vi "Write Sheet3 Data.vi"(0 "Cal Path":path, 5 "Actual Table 1":string[][](array[string]), 7 "Dev Table 1":string[][](array[string]), 9 "Dev Table 2":string[][](array[string]), 11 "Cal Point":i32) -> ()   [LabVIEW 2013]
uses:
  Type Defs/Excel Driver Operator Type Def.ctl
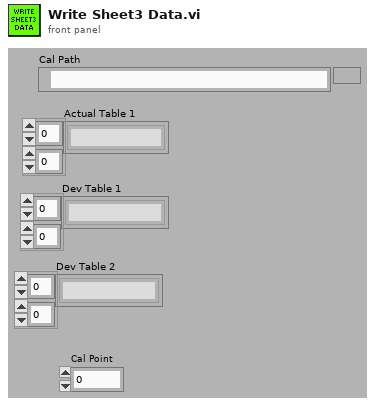
[diagram p1: front panel]
types:
  T1 = typedef "Excel Driver Operator Type Def.ctl" = enum16{"Open", "Close", "Search for String", "GetUsedRange", "Read Range", "Read Cell", "Set Range", "Set Cell"}
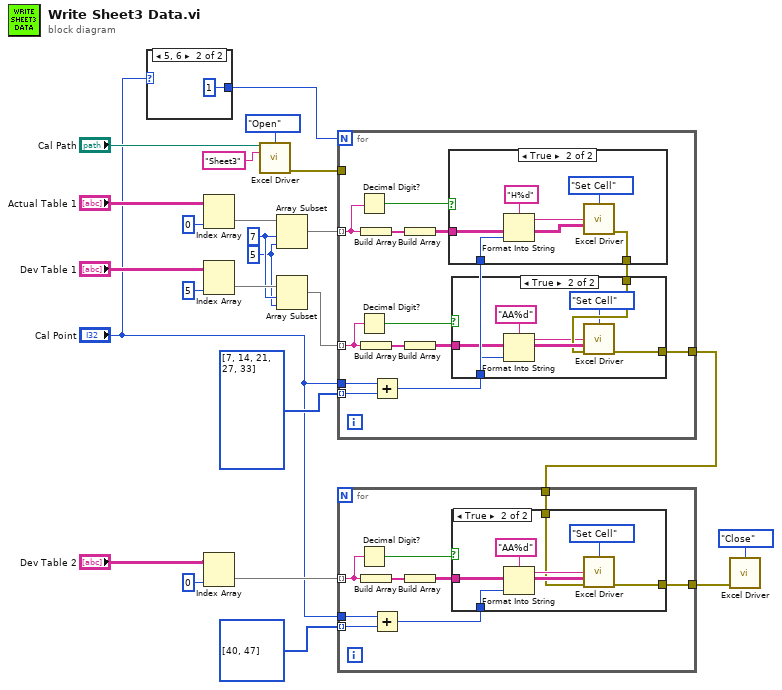
[diagram p0: block diagram]
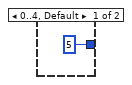
[diagram p2: hidden frame]
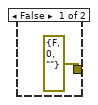
[diagram p3: hidden frame]
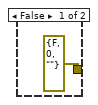
[diagram p4: hidden frame]
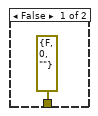
[diagram p5: hidden frame]
diagram:
  w12 = 5 ("length")
  w13 = 7 ("index")
  n1 = case shown="5, 6" "Cal Point" {
    tunnel: [5 1] -> w1
    frame 0..4, Default {
    }
    frame 5, 6 {
    }
  }
  n2 = Index Array(array="Actual Table 1", index (col)=0 ("disabled index (col)")) -> (element=w15:string[])  [unwired: 1 in]
  n3 = Index Array(array="Dev Table 1", index (col)=5 ("disabled index (col)")) -> (element=w14:string[])  [unwired: 1 in]
  n4 = Index Array(array="Dev Table 2", index (col)=0 ("disabled index (col)")) -> (element=w6:string[])  [unwired: 1 in]
  n5 = call "Excel Driver.vi"("Filename of Workbook"="Cal Path", "Operator"=Excel_Driver_Operator_Type_Def."Open", "WorkSheet Name"="Sheet3") -> ("error out"=w23:errorcluster)  [unwired: 10 in, 2 out]
  n6 = Array Subset(array=w15, index=w13, length=w12) -> (w11:string[])
  n7 = Array Subset(array=w14, index=w13, length=w12) -> (w10:string[])
  n8 = for {
    N: w1 -> [_]
    tunnel: w11 -> [w30] mode=indexing
    tunnel: w10 -> [w28] mode=indexing
    tunnel: w23 -> [_]
    tunnel: [w34] -> w4
    tunnel: "Cal Point" -> [w33]
    tunnel: i32[] [7, 14, 21, 27, 33] -> [w32] mode=indexing
    n9 = Decimal Digit?(1:w30) -> (0:w29:bool)
    n10 = Decimal Digit?(1:w28) -> (0:w27:bool)
    n11 = Build Array(w30) -> (w39:string[])
    n12 = Build Array(w28) -> (w37:string[])
    n13 = Add(x=w33, y=w32) -> (x+y=w31:i32)
    n14 = Build Array(w39) -> (w38:string[][])
    n15 = Build Array(w37) -> (w36:string[][])
    n16 = case shown="True" w29 {
      tunnel: w38 -> [_ w53]
      tunnel: [errorcluster {"status"=FALSE, "code"=0, "source"=""} ("error out") w51] -> w35
      tunnel: w31 -> [_ w49]
      frame False {
      }
      frame True {
        n17 = Format Into String(format string="H%d", w49) -> (resulting string=w50:string)  [unwired: 2 in, 1 out]
        n18 = call "Excel Driver.vi"("Operator"=Excel_Driver_Operator_Type_Def."Set Cell", "Range String\n(Or Search String)"=w50, "Cell Values INPUT"=w53) -> ("error out"=w51:errorcluster)  [unwired: 10 in, 2 out]
      }
    }
    n19 = case shown="True" w27 {
      tunnel: w36 -> [_ w46]
      tunnel: w35 -> [_ w45]
      tunnel: [errorcluster {"status"=FALSE, "code"=0, "source"=""} ("error out") w44] -> w34
      tunnel: w31 -> [_ w42]
      frame False {
      }
      frame True {
        n20 = Format Into String(format string="AA%d", w42) -> (resulting string=w43:string)  [unwired: 2 in, 1 out]
        n21 = call "Excel Driver.vi"("Operator"=Excel_Driver_Operator_Type_Def."Set Cell", "Range String\n(Or Search String)"=w43, "Cell Values INPUT"=w46, "error in (no error)"=w45) -> ("error out"=w44:errorcluster)  [unwired: 9 in, 2 out]
      }
    }
  }
  n22 = for {
    tunnel: w6 -> [w57] mode=indexing
    tunnel: [w61] -> w3
    tunnel: "Cal Point" -> [w60]
    tunnel: i32[] [40, 47] -> [w59] mode=indexing
    tunnel: w4 -> [w55]
    n23 = Decimal Digit?(1:w57) -> (0:w56:bool)
    n24 = Build Array(w57) -> (w63:string[])
    n25 = Add(x=w60, y=w59) -> (x+y=w58:i32)
    n26 = Build Array(w63) -> (w62:string[][])
    n27 = case shown="True" w56 {
      tunnel: w62 -> [_ w70]
      tunnel: [errorcluster {"status"=FALSE, "code"=0, "source"=""} ("error out") w69] -> w61
      tunnel: w58 -> [_ w67]
      tunnel: w55 -> [_ w65]
      frame False {
      }
      frame True {
        n28 = Format Into String(format string="AA%d", w67) -> (resulting string=w68:string)  [unwired: 2 in, 1 out]
        n29 = call "Excel Driver.vi"("Operator"=Excel_Driver_Operator_Type_Def."Set Cell", "Range String\n(Or Search String)"=w68, "Cell Values INPUT"=w70, "error in (no error)"=w65) -> ("error out"=w69:errorcluster)  [unwired: 9 in, 2 out]
      }
    }
  }
  n30 = call "Excel Driver.vi"("Operator"=Excel_Driver_Operator_Type_Def."Close", "error in (no error)"=w3) -> ()  [unwired: 11 in, 3 out]
